vi "数组.vi"() -> ()   [LabVIEW 2020]
panel:
  out "数组 5":dbl[](array[numeric])
  out "数组子集":dbl[][](array[numeric])
  in  "2维数组":dbl[][](array[numeric])
  out "数组 4":dbl[][](array[numeric])
  out "数组 3":dbl[][](array[numeric])
  in  "2维数组 2":dbl[][](array[numeric])
  out "数组 2":dbl[][](array[numeric])
  in  "插入元素":dbl[](array[numeric])
  in  "2维数组":dbl[][](array[numeric])
  out "数组":dbl[][](array[numeric])
  in  "1维数组":dbl[](array[numeric])
  in  "替换子集":dbl[][](array[numeric])
  out "数值":dbl
  in  "索引数组":dbl[][](array[numeric])
  out "二维数组大小":dbl[](array[numeric])
  in  "1维数组":dbl[](array[numeric])
  out "一维数组大小":dbl
  in  "2维数组":dbl[][](array[numeric])
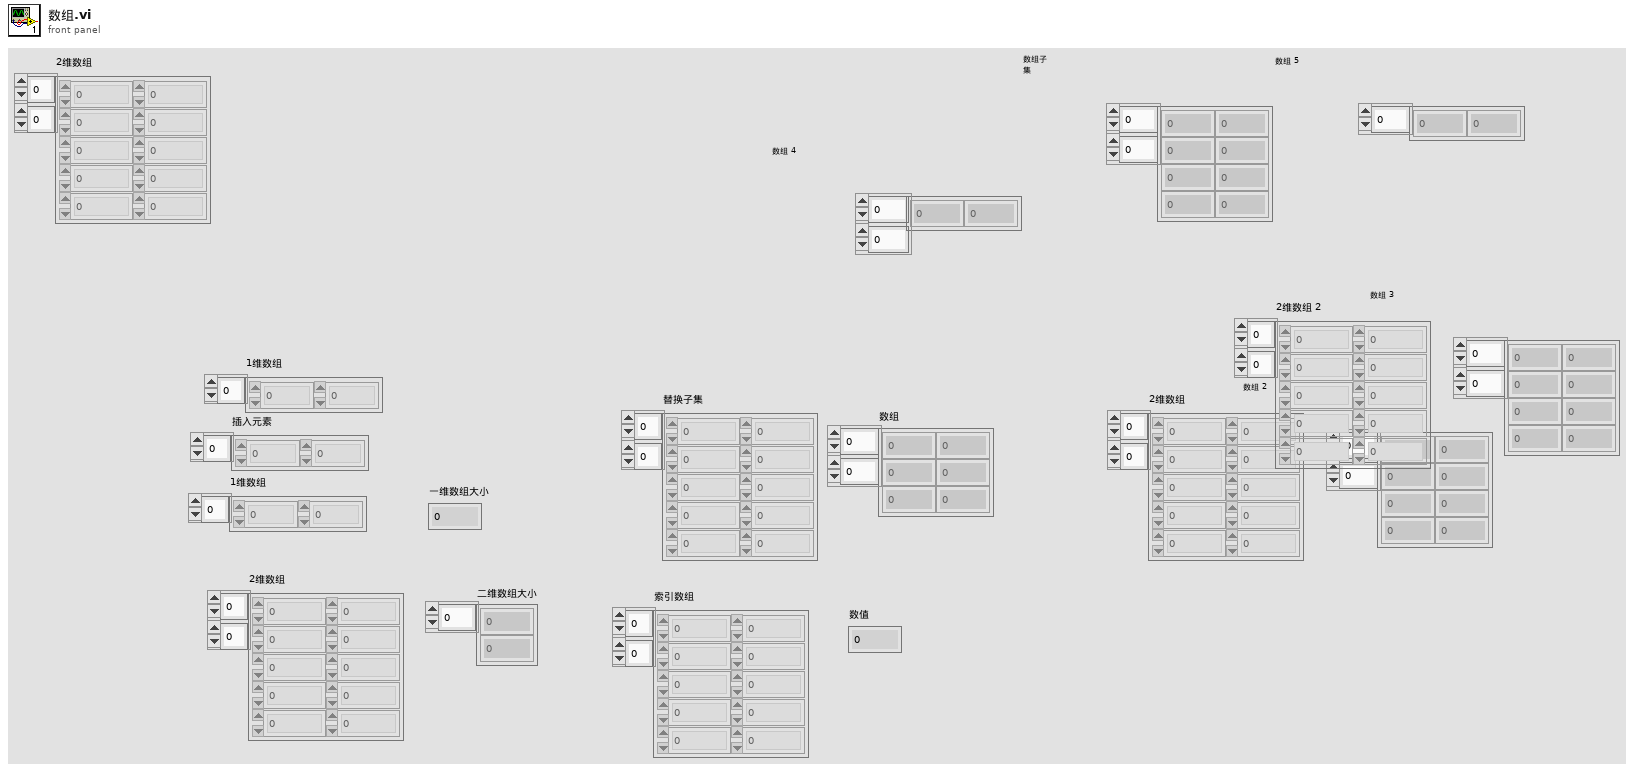
[diagram p1: front panel]
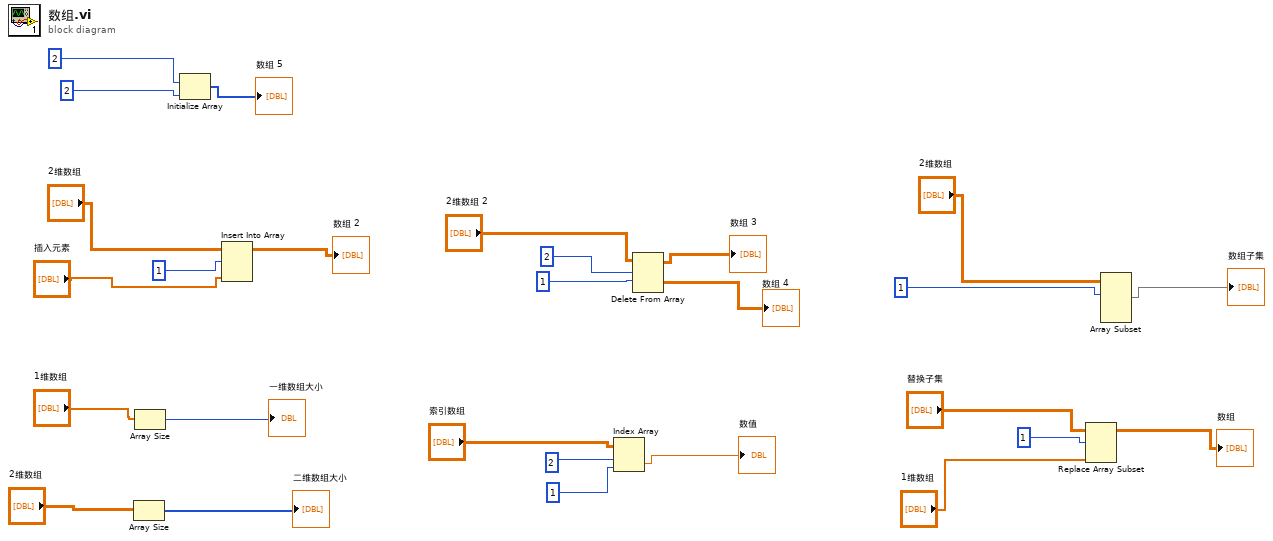
[diagram p0: block diagram]
diagram:
  n1 = Array Size(array="2维数组") -> (size(s)=→"二维数组大小":i32[])
  n2 = Array Size(array="1维数组") -> (size(s)=→"一维数组大小":i32)
  n3 = Initialize Array(2, 2) -> (→"数组 5":i32[])
  n4 = Insert Into Array(array="2维数组", index (row)=1, new element="插入元素") -> (→"数组 2":dbl[][])  [unwired: 1 in]
  n5 = Index Array(array="索引数组", index (row)=2, index (col)=1) -> (element=→"数值":dbl)
  n6 = Delete From Array(array="2维数组 2", length=2, index (row)=1) -> (deleted portion=→"数组 4":dbl[][], array with subset deleted=→"数组 3":dbl[][])  [unwired: 1 in]
  n7 = Replace Array Subset(array="替换子集", new element="1维数组", index (row)=1) -> (→"数组":dbl[][])  [unwired: 1 in]
  n8 = Array Subset(array="2维数组", index (row)=1) -> (→"数组子集":dbl[][])  [unwired: 3 in]
